vi "Convert To JSON Comp Format.vi"(11 "input settings":T2={"number of channels"=51200, "data justification"=enum."Right Justified", "endianness"=enum."MSB First", "channel length"=0, "bit depth"=0, "frame clock rate"=0.0, "bit clock edge sync"=enum."Falling", "master clock source"=enum."Internal", "master clock rate"=0.0, "Logic Level"=enum."1.2 V", "frame sync edge for channel 0"=enum."Rising", "Channel 0 Offset"=0}) -> (3 "input settings JSON":T1={"number of channels"=51200, "data justification"="", "endianness"="", "channel length"=5, "bit depth"=0, "frame clock rate"=0.0, "bit clock edge sync"="", "master clock souce"="", "master clock rate"=0.0, "logic level"="", "frame sync edge for channel 0"="", "Channel 0 Offset"=0})   [LabVIEW 2022 SP3, in "Digital Serial Input Settings.lvlib"]
uses:
  Digital Serial Input Settings.lvlib
  controls/digital serial input settings.ctl
  <vilib>/PDM Acquisition Toolkit/shared/controls/PCM Data Justification.ctl
  <vilib>/PDM Acquisition Toolkit/shared/controls/PCM Bit Endianness.ctl
  <vilib>/PDM Acquisition Toolkit/shared/controls/Digital Edge.ctl
  controls/digital audio protocol/master clock source.ctl
  <vilib>/PDM Acquisition Toolkit/host/Classes/Session/Controls/Logic Levels.ctl
  digital serial input settings_json.ctl
  <vilib>/PDM Acquisition Toolkit/shared/PDM Shared.lvlib
  <vilib>/PDM Acquisition Toolkit/host/Classes/Session/DecoderSession.lvclass
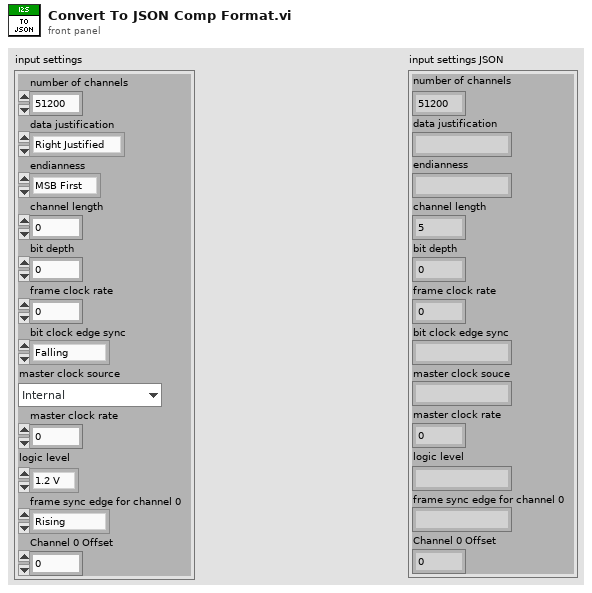
[diagram p1: front panel]
types:
  T1 = typedef "Digital Serial Input Settings.lvlib/digital serial input settings_json.ctl" = cluster{"number of channels":u32, "data justification":string, "endianness":string, "channel length":u32, "bit depth":u32, "frame clock rate":dbl, "bit clock edge sync":string, "master clock souce":string, "master clock rate":dbl, "logic level":string, "frame sync edge for channel 0":string, "Channel 0 Offset":u32}
  T2 = typedef "digital serial input settings.ctl" = cluster{"number of channels":u32, "data justification":T3, "endianness":T4, "channel length":u32, "bit depth":u32, "frame clock rate":dbl, "bit clock edge sync":T5, "master clock source":T6, "master clock rate":dbl, "Logic Level":T7, "frame sync edge for channel 0":T5, "Channel 0 Offset":u32}
  T3 = typedef "PDM Shared.lvlib/PCM Data Justification.ctl" = enum16{"Left Justified", "Right Justified"}
  T4 = typedef "PDM Shared.lvlib/PCM Bit Endianness.ctl" = enum16{"MSB First", "LSB First"}
  T5 = typedef "PDM Shared.lvlib/Digital Edge.ctl" = enum8{"Rising", "Falling"}
  T6 = typedef "master clock source.ctl" = enum32{"Internal", "External"}
  T7 = typedef "PDM Acquisition Class Library.lvlib/DecoderSession.lvclass/Logic Levels.ctl" = enum16{"3.3 V", "1.8 V", "1.2 V"}
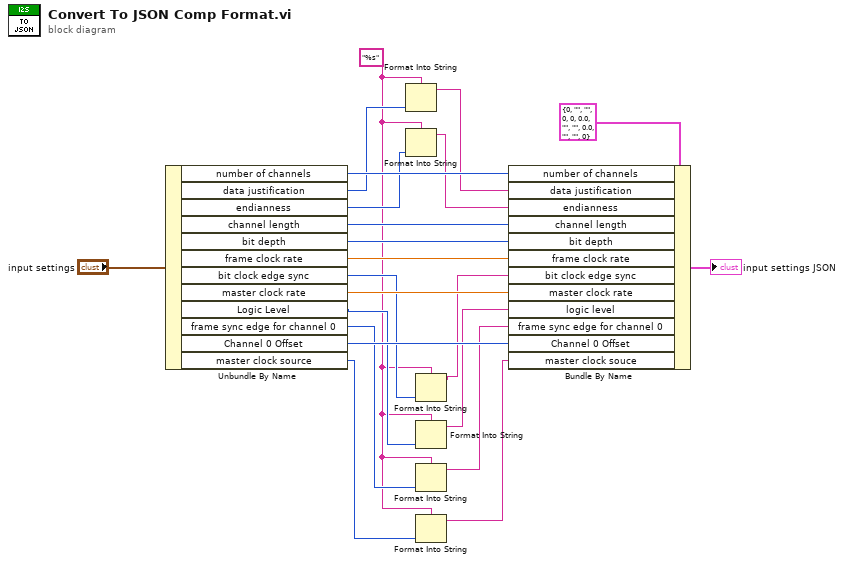
[diagram p0: block diagram]
diagram:
  w4 = "%s" ("format string")
  n1 = Unbundle By Name("input settings") -> ("number of channels"=w21:u32, "data justification"=w15:T3, "endianness"=w13:T4, "channel length"=w20:u32, "bit depth"=w19:u32, "frame clock rate"=w18:dbl, "bit clock edge sync"=w11:T5, "master clock rate"=w17:dbl, "Logic Level"=w10:T7, "frame sync edge for channel 0"=w9:T5, "Channel 0 Offset"=w16:u32, "master clock source"=w5:T6)
  n2 = Format Into String(format string=w4, w15) -> (resulting string=w14:string)  [unwired: 2 in, 1 out]
  n3 = Format Into String(format string=w4, w13) -> (resulting string=w12:string)  [unwired: 2 in, 1 out]
  n4 = Format Into String(format string=w4, w11) -> (resulting string=w7:string)  [unwired: 2 in, 1 out]
  n5 = Format Into String(format string=w4, w10) -> (resulting string=w6:string)  [unwired: 2 in, 1 out]
  n6 = Format Into String(format string=w4, w9) -> (resulting string=w8:string)  [unwired: 2 in, 1 out]
  n7 = Format Into String(format string=w4, w5) -> (resulting string=w3:string)  [unwired: 2 in, 1 out]
  n8 = Bundle By Name(cluster=T1 {"number of channels"=0, "data justification"="", "endianness"="", "channel length"=0, "bit depth"=0, "frame clock rate"=0.0, "bit clock edge sync"="", "master clock souce"="", "master clock rate"=0.0, "logic level"="", "frame sync edge for channel 0"="", "Channel 0 Offset"=0} ("JSON compatible settings"), "number of channels"=w21, "data justification"=w14, "endianness"=w12, "channel length"=w20, "bit depth"=w19, "frame clock rate"=w18, "bit clock edge sync"=w7, "master clock rate"=w17, "logic level"=w6, "frame sync edge for channel 0"=w8, "Channel 0 Offset"=w16, "master clock souce"=w3) -> (→"input settings JSON":T1)
